vi "MTM2_logEvent_hardpointList.vi"(8 "error in (no error)":errorcluster, 11 "logevent_hardpointList_Ctl":T1={"private_rcvStamp"=0.0, "actuators[6]"=[0, 0, 0, 0, 0, 0], "priority"=0}) -> (0 "error out":errorcluster, 2 "function return":i32, 3 "logevent_hardpointList_Ctl out":T1)   [LabVIEW 2018, in "SALLV_MTM2.lvlib"]
doc: "int MTM2_shm_logEvent_hardpointListLV(MTM2_logevent_hardpointListLV *logevent_hardpointList_Ctl );"
uses:
  DataTypes/logevent_hardpointList.ctl
  SALLV_MTM2.lvlib
  SALLV_MTM2.so
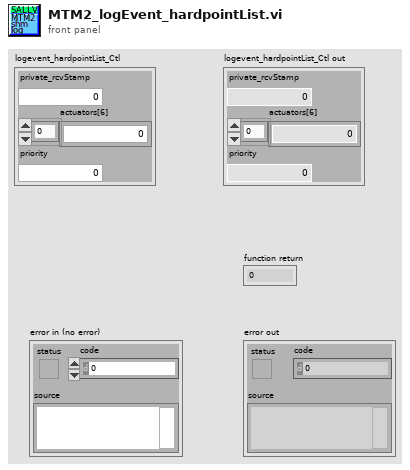
[diagram p1: front panel]
types:
  T1 = typedef "SALLV_MTM2.lvlib/logevent_hardpointList.ctl" = cluster{"private_rcvStamp":dbl, "actuators[6]":u16[], "priority":i32}
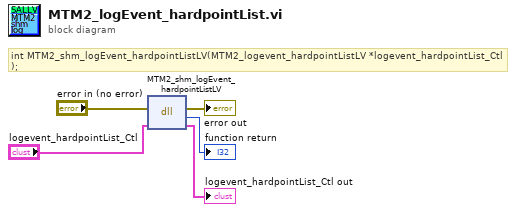
[diagram p0: block diagram]
diagram:
  # "int MTM2_shm_logEvent_hardpointListLV(MTM2_logevent_hardpointListLV *logevent_hardpointList_Ctl );"
  n1 = dll-call lib="home/ttsai/Documents/salLabviewApi/SALLV_MTM2/SALLV_MTM2.*" fn="MTM2_shm_logEvent_hardpointListLV"(error in="error in (no error)", "logevent_hardpointList_Ctl"="logevent_hardpointList_Ctl") -> (error out=→"error out":errorcluster, →"function return":i32, "logevent_hardpointList_Ctl"=→"logevent_hardpointList_Ctl out":T1)  [unwired: 2 in, 1 out]
